vi "session_get_data.vi"(8 "error in":errorcluster, 11 "VISA resource name":refnum<visa-resource-name>) -> (0 "error out":errorcluster, 2 "Session User Data out":T1={"Instr type"="", "Instr type for err. msg."="", "Installed Options"=[], "OPC Timeout"=5000, "Query Instrument Status"=TRUE, "Check Range"=TRUE, "Check Options"=TRUE, "Add LF to Write"=TRUE, "Simulate"=FALSE, "Logging"=FALSE, "Logging params"=variant, "Interface Type"=enum."GPIB_VXI", "Fast Sweep"=0, "AdditionalFlags"=0, "WaitBeforeWrite"=5000, "WaitBeforeRead"=0, "BinDataChunkSize"=0} {"BinDataChunkSize" format="%.0p"; "AdditionalFlags" format="%08b"; "Fast Sweep" items=["Normal", "Fast"]}, 3 "VISA resource name out":refnum<visa-resource-name> caption="VISA resource name")   [LabVIEW 2014, in "rszvl_rsidr_core.lvlib"]
uses:
  rszvl_rsidr_core.lvlib
  type_Session_Data.ctl
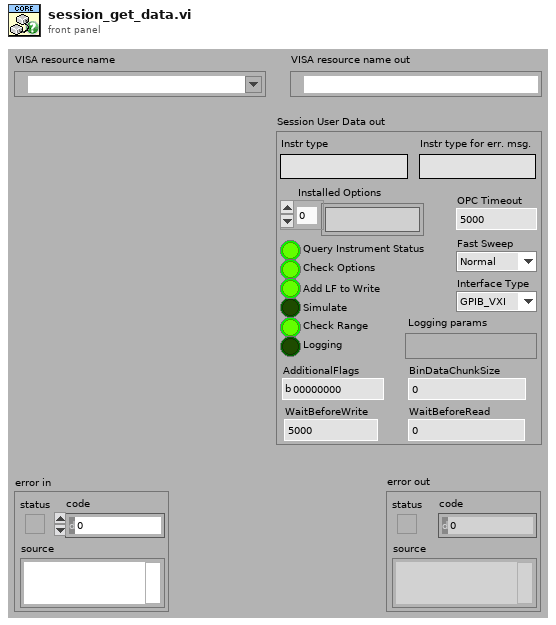
[diagram p1: front panel]
types:
  T1 = typedef "rszvl_rsidr_core.lvlib/type_Session_Data.ctl" = cluster{"Instr type":string, "Instr type for err. msg.":string, "Installed Options":string[], "OPC Timeout":i32, "Query Instrument Status":bool, "Check Range":bool, "Check Options":bool, "Add LF to Write":bool, "Simulate":bool, "Logging":bool, "Logging params":variant, "Interface Type":enum16{"Unknown", "GPIB", "VXI", "GPIB_VXI", "ASRL", "PXI", "TCPIP", "USB", "SOCKET"}, "Fast Sweep":i32, "AdditionalFlags":i32, "WaitBeforeWrite":i32, "WaitBeforeRead":i32, "BinDataChunkSize":i64}
  T2 = enum16{"Initialize", "GetData", "SetData", "Clear"}
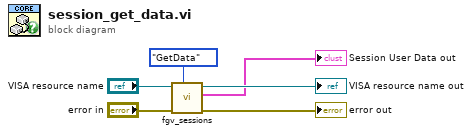
[diagram p0: block diagram]
diagram:
  n1 = call "fgv_sessions.vi"("Operation"=T2."GetData", "error in"="error in", "VISA resource name"="VISA resource name") -> ("error out"=→"error out":errorcluster, "Session User Data out"=→"Session User Data out":T1, "VISA resource name out"=→"VISA resource name out":refnum<visa-resource-name>)  [unwired: 6 in]
